vi "Afisare3D3_2020.vi"() -> ()   [LabVIEW 2016]
uses:
  <vilib>/Utility/miscctls.llb/LVRGBAColorTypeDef.ctl
  <vilib>/Instr/_visa.llb/VISA Configure Serial Port (Instr).vi
  <vilib>/picture/3D Picture Control/Object/Create Object (drawable).vi
  <vilib>/picture/3D Picture Control/Helpers/Apply Texture (no reference).vi
  <vilib>/picture/3D Picture Control/NI_3D Picture Control.lvlib
panel:
  in  "Filter Mode":T1(ring)=enum."Linear Filtration"
  out "Numeric 2":dbl
  out "Numeric":dbl
  in  "Background Color":T2={"Red"=0.5, "Green"=0.8, "Blue"=1.0, "Alpha"=0.0}
  out "String":string
  in  "VISA resource name":refnum<visa-resource-name>
  in  "X":i8(knob)=-6 scale=-50.0..100.0
  in  "stop":bool
  out "3D Picture":refnum<vi>(3d-picture)
  in  "Y":i8(knob)=-31 scale=-50.0..100.0
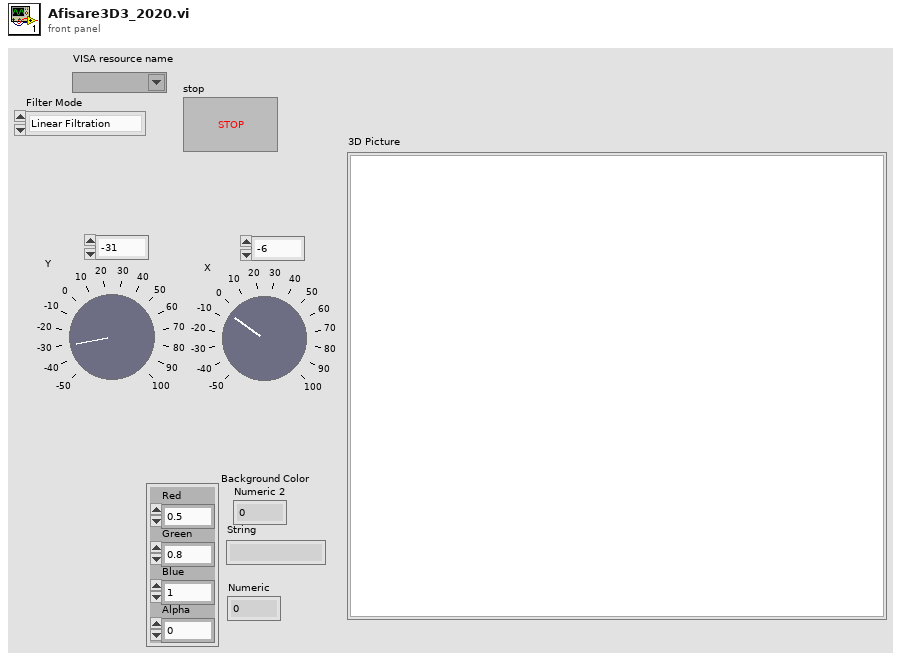
[diagram p1: front panel]
types:
  T1 = enum16{"No Filtration", "Linear Filtration", "Simple Mipmap Filtration", "Bilinear Filtration", "Trilinear Filtration"}
  T2 = typedef "LVRGBAColorTypeDef.ctl" = cluster{"Red":sgl, "Green":sgl, "Blue":sgl, "Alpha":sgl}
  T3 = typedef "imagedata.ctl" = cluster{"image type":i32, "image depth":i32, "image":u8[], "mask":u8[], "colors":u32[], "Rectangle":cluster{"left":i16, "top":i16, "right":i16, "bottom":i16}}
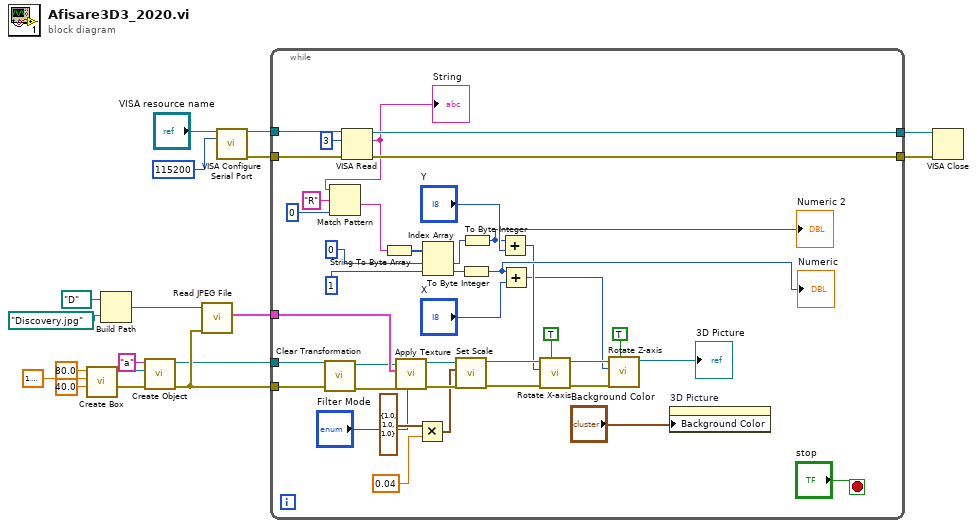
[diagram p0: block diagram]
diagram:
  n1 = call <vilib>:"Create Box.vi"("Length Z"=sgl 40.0, "Length Y"=sgl 1.2, "Length X"=sgl 80.0) -> ("error out"=w9:errorcluster, "New Box Refnum"=w4:refnum<vi>)  [unwired: 7 in]
  n2 = Build Path(base path=path "D:/", name or relative path=path "Discovery.jpg" ("Name")) -> (appended path=w10:path)
  n3 = call-poly <vilib>:"Create Object.vi"("error in (no error)"=w9, "Geometry"=w4, "Name"="a") -> ("error out"=w3:errorcluster, "Scene:New Object"=w2:refnum<vi>)  [unwired: 7 in]
  n4 = call <vilib>:"Read JPEG File.vi"("error in (no error)"=w3, "path to JPEG file"=w10) -> ("image data"=w1:T3)  [unwired: 7 in, 2 out]
  n5 = call-poly "VISA Configure Serial Port"("VISA resource name"="VISA resource name", "baud rate (9600)"=u32 115200) -> ("VISA resource name out"=w18:refnum<visa-resource-name>, "error out"=w16:errorcluster)  [unwired: 12 in]
  n6 = while {
    tunnel: w18 -> [w48]
    tunnel: [w47] -> w17
    tunnel: w16 -> [w46]
    tunnel: [w45] -> w15
    tunnel: w3 -> [w32]
    tunnel: w2 -> [w34]
    tunnel: w1 -> [w43]
    stop <- "stop" stop-if-true
    n7 = call <vilib>:"Clear Transformation.vi"("error in (no error)"=w32, "Object Refnum In"=w34) -> ("error out"=w31:errorcluster, "Object Refnum Out"=w33:refnum<vi>)  [unwired: 8 out]
    n8 = VISA Read(VISA resource name=w48, byte count=u32 3, error in (no error)=w46) -> (VISA resource name out=w47:refnum<visa-resource-name>, read buffer=w25:string, error out=w45:errorcluster)  [unwired: 1 out]
    "String" <- w25
    n9 = Match Pattern(string=w25, regular expression="R", offset (0)=0) -> (after substring=w26:string)  [unwired: 3 out]
    n10 = String To Byte Array(string=w26) -> (unsigned byte array=w38:u8[])
    n11 = call-poly <vilib>:"Apply Texture.vi"("Filter Mode"="Filter Mode", "error in (no error)"=w31, "Image Data"=w43, "Scene Object In"=w33) -> ("error out"=w50:errorcluster, "Scene Object Out"=w49:refnum<vi>)  [unwired: 6 in]
    n12 = Multiply(x=cluster{"X":sgl, "Y":sgl, "Z":sgl} {"X"=1.0, "Y"=1.0, "Z"=1.0} ("Scale"), y=0.04) -> (x*y=w41:cluster{"X":dbl, "Y":dbl, "Z":dbl})
    n13 = Index Array "Index Array"(array=w38, index #1=0 ("index"), index #2=1 ("index")) -> (element #1=w35:u8, element #2=w36:u8)
    n14 = call <vilib>:"Set Scale.vi"("error in (no error)"=w50, "Scale"=w41, "Scene Object"=w49) -> ("error out"=w52:errorcluster, "Scaled Object"=w51:refnum<vi>)  [unwired: 7 in]
    n15 = To Byte Integer(number=w36) -> (8bit integer=w22:i8)
    "Numeric" <- w22
    n16 = To Byte Integer(number=w35) -> (8bit integer=w23:i8)
    "Numeric 2" <- w23
    n17 = Add(x=w23, y="Y") -> (x+y=w20:i8)
    n18 = Add(x=w22, y="X") -> (x+y=w19:i8)
    n19 = call <vilib>:"Rotate X-axis.vi"("Relative?"=TRUE, "error in (no error)"=w52, "angle"=w20, "Scene Object In"=w51) -> ("error out"=w57:errorcluster, "Scene Object Out"=w56:refnum<vi>)  [unwired: 6 in]
    n20 = call <vilib>:"Rotate Z-axis.vi"("Relative?"=TRUE, "error in (no error)"=w57, "angle"=w19, "Scene Object In"=w56) -> ("Scene Object Out"=→"3D Picture":refnum<vi>)  [unwired: 6 in, 1 out]
    n21 = property on="3D Picture" class="SceneGraphDisp (strict)"("Background Color"="Background Color") -> ()  [unwired: 2 in, 2 out]
  }
  n22 = VISA Close(VISA resource name=w17, error in (no error)=w15) -> ()  [unwired: 1 out]
